vi "Create Data Folders.vi"(10 "Experiment Indicator":string, 11 "username":string) -> (3 "Data Output Folder":path)   [LabVIEW 2011]
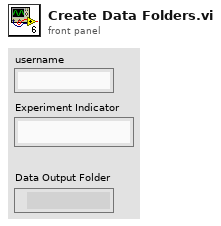
[diagram p1: front panel]
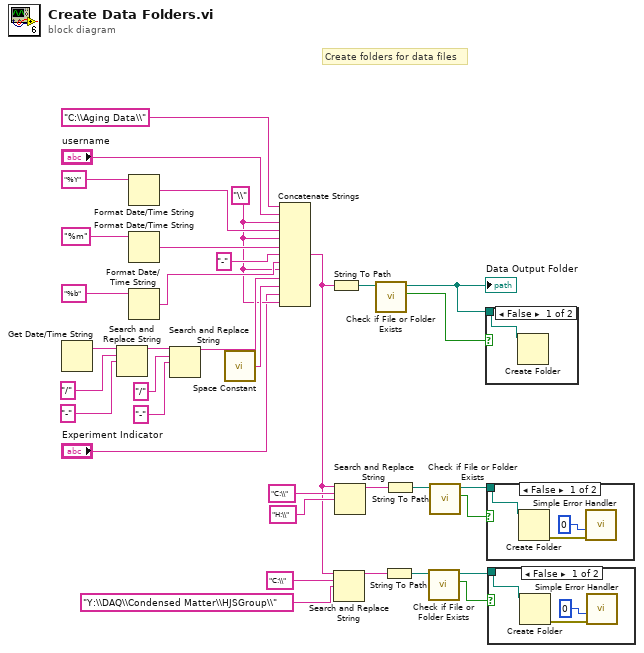
[diagram p0: block diagram]
diagram:
  w10 = "\\"
  # "Create folders for data files"
  n1 = Get Date/Time String() -> (date string=w23:string)  [unwired: 3 in, 1 out]
  n2 = Search and Replace String(input string=w23, search string="/", replace string="-") -> (result string=w13:string)  [unwired: 5 in, 3 out]
  n3 = Format Date/Time String(time format string (%c)="%Y") -> (date/time string=w29:string)  [unwired: 2 in]
  n4 = Format Date/Time String(time format string (%c)="%m") -> (date/time string=w28:string)  [unwired: 2 in]
  n5 = Format Date/Time String(time format string (%c)="%b") -> (date/time string=w27:string)  [unwired: 2 in]
  n6 = Search and Replace String(input string=w13, search string="/", replace string="-") -> (result string=w12:string)  [unwired: 5 in, 3 out]
  n7 = call <vilib>:"Space Constant.vi"() -> ("String"=w11:string)
  n8 = Concatenate Strings("C:\\Aging Data\\", "username", w10, w29, w10, w28, "-", w27, w10, w12, w11, "Experiment Indicator", w10) -> (w6:string)
  n9 = String To Path(string=w6) -> (path=w34:path)
  n10 = Search and Replace String(input string=w6, search string="C:\\", replace string="Y:\\DAQ\\Condensed Matter\\HJSGroup\\") -> (result string=w16:string)  [unwired: 5 in, 3 out]
  n11 = Search and Replace String(input string=w6, search string="C:\\", replace string="H:\\") -> (result string=w20:string)  [unwired: 5 in, 3 out]
  n12 = call <vilib>:"Check if File or Folder Exists.vi"("path"=w34) -> ("file or folder exists?"=w35:bool, "dup path"=w1:path)  [unwired: 8 in, 1 out]
  "Data Output Folder" <- w1
  n13 = String To Path(string=w16) -> (path=w24:path)
  n14 = String To Path(string=w20) -> (path=w25:path)
  n15 = call <vilib>:"Check if File or Folder Exists.vi"("path"=w24) -> ("file or folder exists?"=w2:bool, "dup path"=w3:path)  [unwired: 8 in, 1 out]
  n16 = call <vilib>:"Check if File or Folder Exists.vi"("path"=w25) -> ("file or folder exists?"=w4:bool, "dup path"=w5:path)  [unwired: 8 in, 1 out]
  n17 = case shown="False" w35 {
    tunnel: w1 -> [w36 _]
    frame False {
      n18 = Create Folder(path (use dialog)=w36) -> ()  [unwired: 2 in, 3 out]
    }
    frame True {
    }
  }
  n19 = case shown="False" w4 {
    tunnel: w5 -> [w39 _]
    frame False {
      n20 = Create Folder(path (use dialog)=w39) -> (error out=w38:errorcluster)  [unwired: 2 in, 2 out]
      n21 = call <vilib>:"Simple Error Handler.vi"("type of dialog (OK msg:1)"=0, "error in (no error)"=w38) -> ()  [unwired: 3 in, 5 out]
    }
    frame True {
    }
  }
  n22 = case shown="False" w2 {
    tunnel: w3 -> [w42 _]
    frame False {
      n23 = Create Folder(path (use dialog)=w42) -> (error out=w41:errorcluster)  [unwired: 2 in, 2 out]
      n24 = call <vilib>:"Simple Error Handler.vi"("type of dialog (OK msg:1)"=0, "error in (no error)"=w41) -> ()  [unwired: 3 in, 5 out]
    }
    frame True {
    }
  }
